vi "users copy user.vi"(8 "error in (no error)":errorcluster, 9 "All Users (empty)":T1[](array[typedef]), 11 "sxUsername (\"\")":string) -> (0 "error out":errorcluster, 1 "User Information":T1)   [LabVIEW 2011]
uses:
  server/database/Users/User Record.ctl
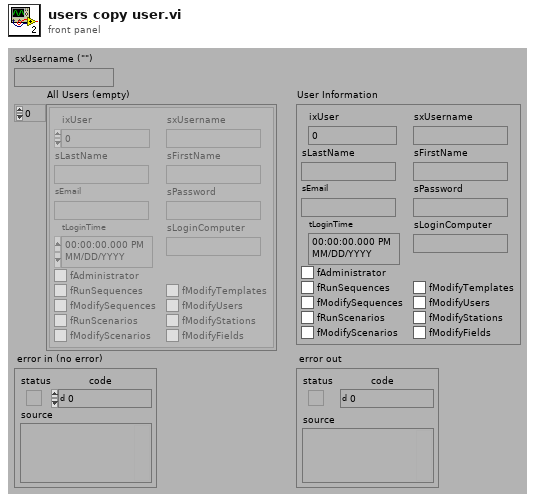
[diagram p1: front panel]
types:
  T1 = typedef "User Record.ctl" = cluster{"ixUser":i32, "sxUsername":string, "sLastName":string, "sFirstName":string, "sEmail":string, "sPassword":string, "tLoginTime":timestamp, "sLoginComputer":string, "fAdministrator":bool, "fRunSequences":bool, "fModifySequences":bool, "fRunScenarios":bool, "fModifyScenarios":bool, "fModifyTemplates":bool, "fModifyUsers":bool, "fModifyStations":bool, "fModifyFields":bool}
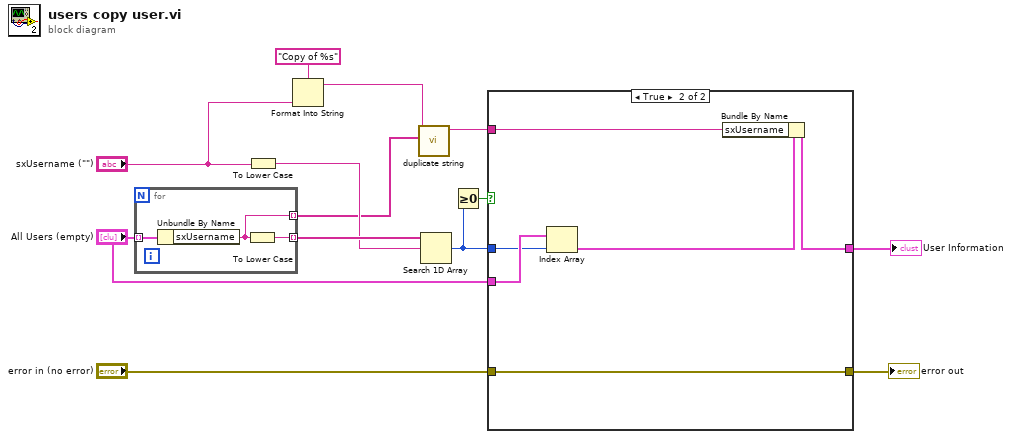
[diagram p0: block diagram]
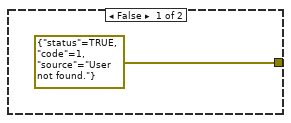
[diagram p2: hidden frame]
diagram:
  n1 = for {
    tunnel: "All Users (empty)" -> [w16] mode=indexing
    tunnel: [w15] -> w13 mode=indexing
    tunnel: [w14] -> w5 mode=indexing
    n2 = Unbundle By Name(w16) -> ("sxUsername"=w14:string)
    n3 = To Lower Case(string=w14) -> (all lower case string=w15:string)
  }
  n4 = To Lower Case(string="sxUsername (\"\")") -> (all lower case string=w12:string)
  n5 = Format Into String(format string="Copy of %s", "sxUsername (\"\")") -> (resulting string=w2:string)  [unwired: 2 in, 1 out]
  n6 = call "duplicate string.vi"("Array of Strings"=w5, "String"=w2) -> ("Updated String"=w1:string)  [unwired: 9 out]
  n7 = Search 1D Array(1D array=w13, element=w12) -> (index of element=w10:i32)  [unwired: 1 out]
  n8 = Greater Or Equal To 0?(x=w10) -> (x >= 0?=w9:bool)
  n9 = case shown="True" w9 {
    tunnel: "All Users (empty)" -> [_ w23]
    tunnel: w10 -> [_ w22]
    tunnel: [_ w19] -> w8
    tunnel: "error in (no error)" -> [_ w21]
    tunnel: [errorcluster {"status"=TRUE, "code"=1, "source"="User not found."} ("error in (no error)") w21] -> w6
    tunnel: w1 -> [_ w18]
    frame False {
    }
    frame True {
      n10 = Index Array(array=w23, index=w22) -> (element=w20:T1)
      n11 = Bundle By Name(cluster=w20, "sxUsername"=w18) -> (w19:T1)
    }
  }
  "error out" <- w6
  "User Information" <- w8
